vi "PicoReadPicoMultiBuffers.vi"(1 "enabled array":i16[](array[numeric]), 2 "Buffer and Transfer Settings":T3={"startIndex"=0, "Samples"=1000000, "Down Sample Ratio"=1, "Down-Sample Mode"=2147483648} {"Down-Sample Mode" items=["None"=2147483648, "Aggregate"=1, "Decimate"=2, "Average"=4]; "Down Sample Ratio" step=1; "Samples" format="%_6p"}, 3 "Variant":string, 5 "Data Pointers":T1, 9 "No of Buffers":i32=1, 11 "error in (no error)":errorcluster) -> (6 "MultiBuffers (Max or non-aggregated)":T2(array[cluster]), 8 "Min Buffers":T2(array[cluster]), 15 "error out":errorcluster)   [LabVIEW 2020]
doc: "Read data from Picodata buffers for Block and 6000a streaming examples"
uses:
  PicoBuffers.ctl
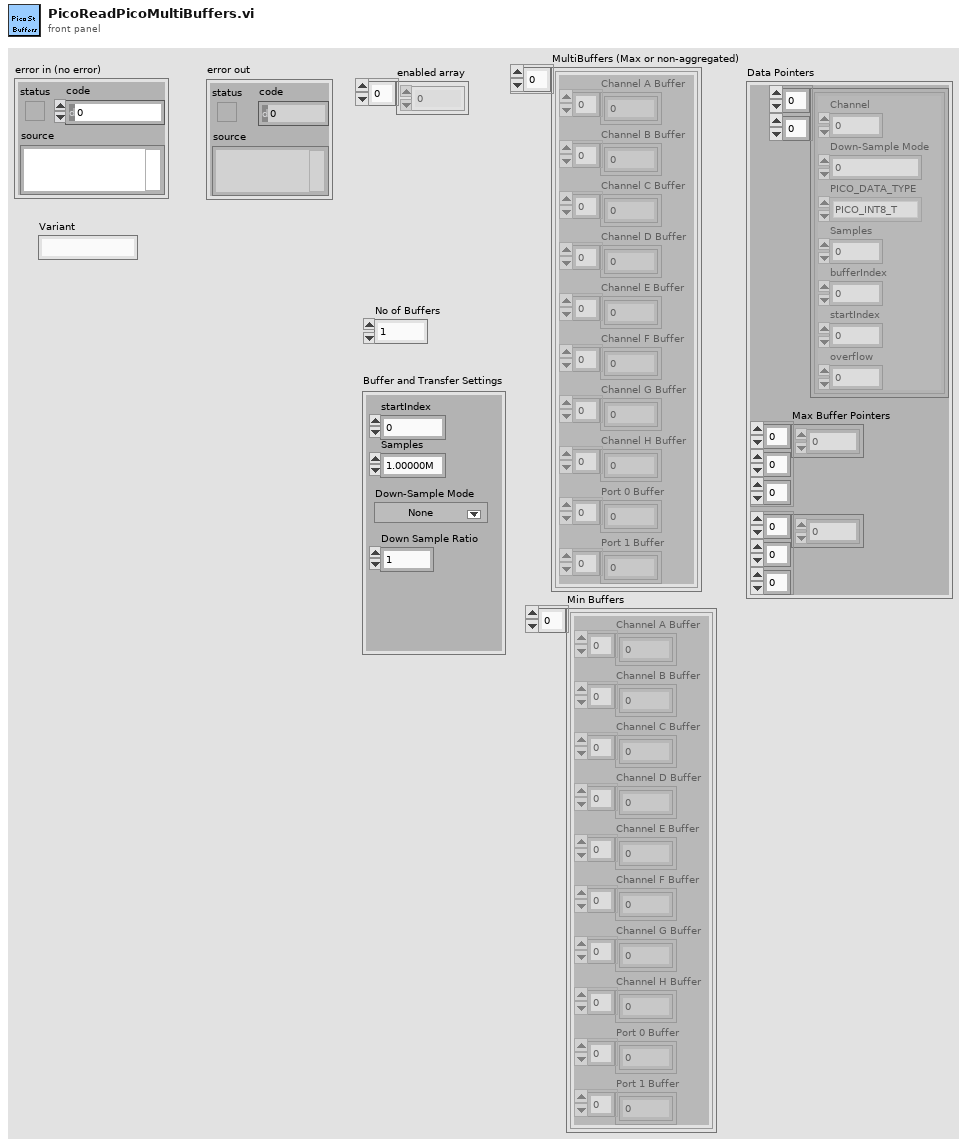
[diagram p1: front panel]
types:
  T1 = typedef "PicoBuffers.ctl" = cluster{"Max Buffer Pointers":u64[][][], "Min Buffer Pointers":u64[][][], "StreamingDataInfo":cluster{"Channel":u32, "Down-Sample Mode":u32, "PICO_DATA_TYPE":enum32{"PICO_INT8_T", "PICO_INT16_T", "PICO_INT32_T", "PICO_UINT32_T", "PICO_INT64_T", ""}, "Samples":i32, "bufferIndex":u64, "startIndex":i32, "overflow":i16}[][]}
  T2 = cluster{"Channel A Buffer":i16[], "Channel B Buffer":i16[], "Channel C Buffer":i16[], "Channel D Buffer":i16[], "Channel E Buffer":i16[], "Channel F Buffer":i16[], "Channel G Buffer":i16[], "Channel H Buffer":i16[], "Port 0 Buffer":i16[], "Port 1 Buffer":i16[]}[]
  T3 = cluster{"startIndex":u64, "Samples":u64, "Down Sample Ratio":u64, "Down-Sample Mode":u32}
  T4 = cluster{"Channel A Buffer":i16[], "Channel B Buffer":i16[], "Channel C Buffer":i16[], "Channel D Buffer":i16[], "Channel E Buffer":i16[], "Channel F Buffer":i16[], "Channel G Buffer":i16[], "Channel H Buffer":i16[], "Port 0 Buffer":i16[], "Port 1 Buffer":i16[]}
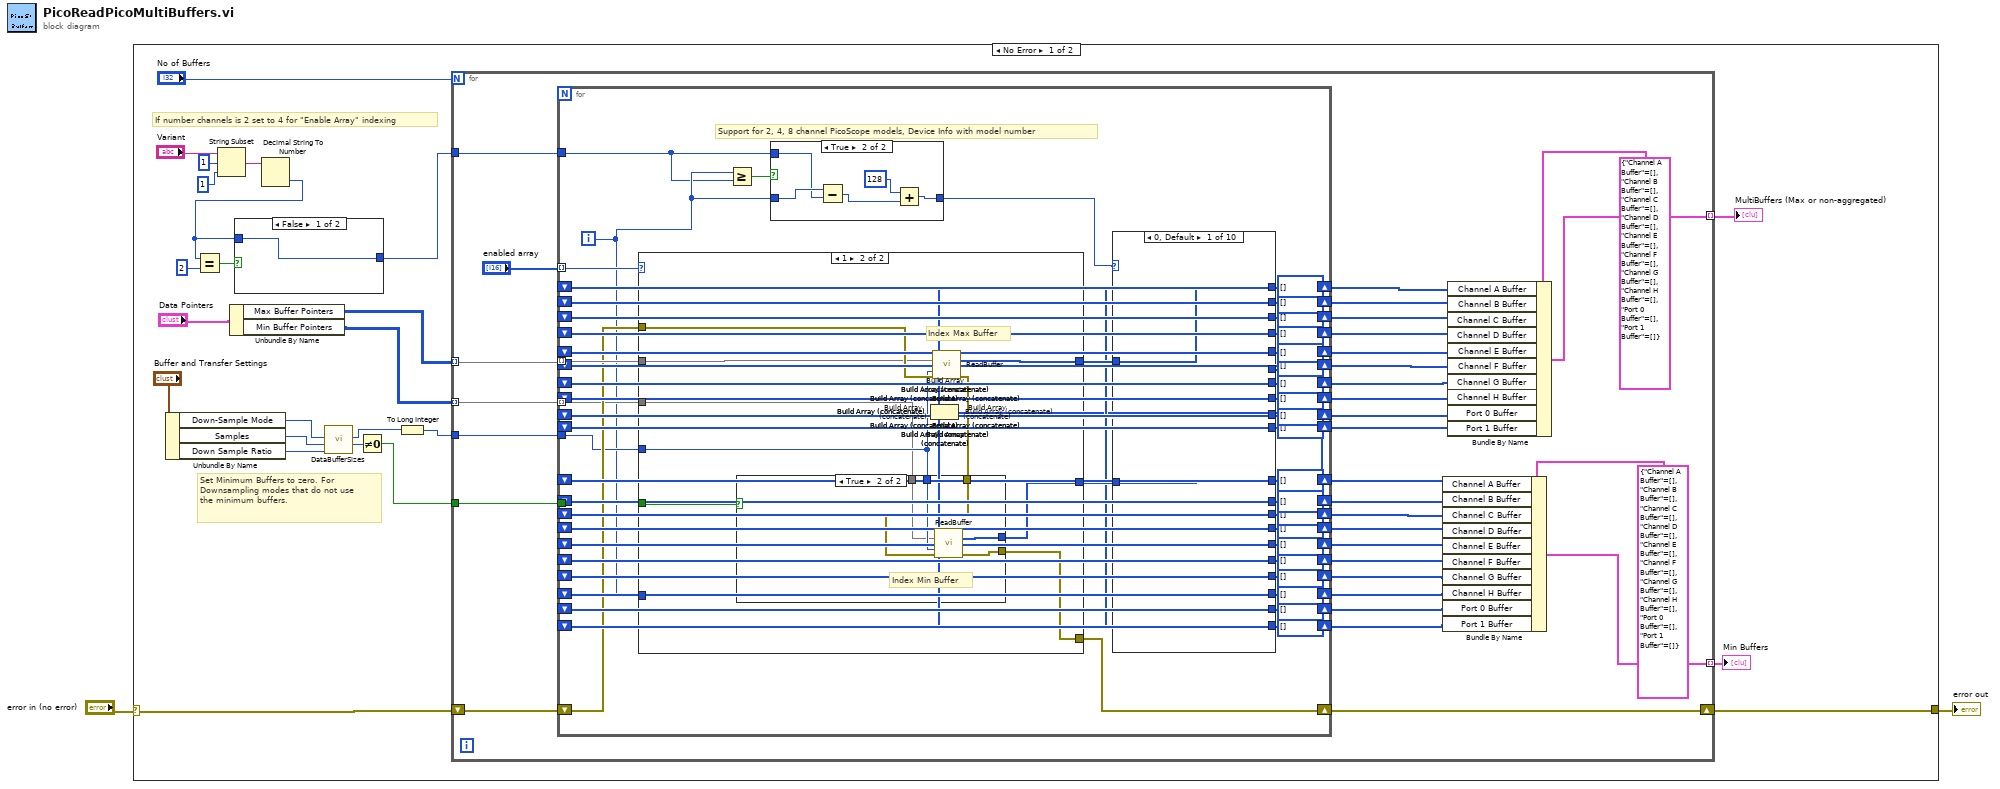
[diagram p0: block diagram]
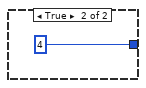
[diagram p2: hidden frame]
diagram:
  n1 = case shown="No Error" "error in (no error)" {
    selector: "error in (no error)" -> [w24 w196]
    tunnel: [w26 w196] -> w1
    frame No Error {
      # "If number channels is 2 set to 4 for \"Enable Array\" indexing"
      # "Set Minimum Buffers to zero. For Downsampling modes that do not use the minimum buffers."
      n2 = Unbundle By Name("Buffer and Transfer Settings") -> ("Down-Sample Mode"=w22:u32, "Samples"=w21:u64, "Down Sample Ratio"=w23:u64)
      n3 = String Subset(string="Variant", offset (0)=1, length (rest)=1 ("length (rest)")) -> (substring=w7:string)
      n4 = Unbundle By Name("Data Pointers") -> ("Max Buffer Pointers"=w12:u64[][][], "Min Buffer Pointers"=w11:u64[][][])
      n5 = Decimal String To Number(string=w7) -> (number=w4:i32)  [unwired: 2 in, 1 out]
      n6 = Equal?(x=w4, y=2 ("Number of channels")) -> (x = y?=w10:bool)
      n7 = case shown="False" w10 {
        tunnel: [w27 4 ("Number of channels")] -> w8
        tunnel: w4 -> [w27 _]
        frame False {
        }
        frame True {
        }
      }
      n8 = call "DataBufferSizes.vi"("Down Sample Ratio"=w23, "Number of Samples"=w21, "Down-Sample Mode"=w22) -> ("min Buffer Size"=w19:i32, "Max Buffer Size"=w15:i32)  [unwired: 7 in]
      n9 = Not Equal To 0?(x=w19) -> (x != 0?=w20:bool)
      n10 = To Long Integer(number=w15) -> (32bit integer=w18:i32)
      n11 = for {
        N: "No of Buffers" -> [_]
        tunnel: [w78] -> w14 mode=indexing
        tunnel: [w77] -> w16 mode=indexing
        tunnel: w20 -> [w65]
        tunnel: w18 -> [w63]
        shift-right: [w80] -> w26
        shift-left: w24 -> [w79]
        tunnel: w12 -> [w61] mode=indexing
        tunnel: w11 -> [w50] mode=indexing
        tunnel: w8 -> [w49]
        n12 = for {
          tunnel: "enabled array" -> [w152] mode=indexing
          tunnel: w61 -> [w153] mode=indexing
          shift-right: [w151] -> w80
          shift-left: w79 -> [w150]
          tunnel: w63 -> [w136]
          tunnel: w65 -> [w135]
          tunnel: w50 -> [w125] mode=indexing
          tunnel: w49 -> [w121]
          shift-right: [w119] -> w76
          shift-left: i16[] [] ("Output Array") -> [w120]
          shift-right: [w117] -> w75
          shift-left: i16[] [] ("Output Array") -> [w118]
          shift-right: [w115] -> w74
          shift-left: i16[] [] ("Output Array") -> [w116]
          shift-right: [w113] -> w73
          shift-left: i16[] [] ("Output Array") -> [w114]
          shift-right: [w111] -> w72
          shift-left: i16[] [] ("Output Array") -> [w112]
          shift-right: [w109] -> w71
          shift-left: i16[] [] ("Output Array") -> [w110]
          shift-right: [w107] -> w64
          shift-left: i16[] [] ("Output Array") -> [w108]
          shift-right: [w105] -> w70
          shift-left: i16[] [] ("Output Array") -> [w106]
          shift-right: [w103] -> w69
          shift-left: i16[] [] ("Output Array") -> [w104]
          shift-right: [w101] -> w68
          shift-left: i16[] [] ("Output Array") -> [w102]
          shift-right: [w99] -> w67
          shift-left: i16[] [] ("Output Array") -> [w100]
          shift-right: [w97] -> w66
          shift-left: i16[] [] ("Output Array") -> [w98]
          shift-right: [w95] -> w58
          shift-left: i16[] [] ("Output Array") -> [w96]
          shift-right: [w93] -> w57
          shift-left: i16[] [] ("Output Array") -> [w94]
          shift-right: [w91] -> w56
          shift-left: i16[] [] ("Output Array") -> [w92]
          shift-right: [w89] -> w55
          shift-left: i16[] [] ("Output Array") -> [w90]
          shift-right: [w87] -> w54
          shift-left: i16[] [] ("Output Array") -> [w88]
          shift-right: [w85] -> w53
          shift-left: i16[] [] ("Output Array") -> [w86]
          shift-right: [w83] -> w52
          shift-left: i16[] [] ("Output Array") -> [w84]
          shift-right: [w81] -> w51
          shift-left: i16[] [] ("Output Array") -> [w82]
          i -> [w122]
          # "Support for 2, 4, 8 channel PicoScope models, Device Info with model number"
          n13 = case shown="1" w152 {
            tunnel: w153 -> [_ w182]
            tunnel: w122 -> [_ _]
            tunnel: [_ w189] -> w149
            tunnel: [_ w188] -> w148
            tunnel: w150 -> [w180 w187]
            tunnel: [w180 w185] -> w151
            tunnel: w136 -> [_ w183]
            tunnel: w135 -> [_ w184]
            tunnel: w125 -> [_ w181]
            frame 0, Default {
            }
            frame 1 {
              # "Index Max Buffer"
              n14 = call "ReadBuffer.vi"("Pointer and BufferSize"=w182, "Buffer size"=w183, "error in (no error)"=w187) -> ("Output Array"=w189:i16[], "error out"=w186:errorcluster)  [unwired: 11 in]
              n15 = case shown="True" w184 {
                tunnel: [_ w195] -> w188
                tunnel: w186 -> [w190 w194]
                tunnel: [w190 w193] -> w185
                tunnel: w183 -> [_ w192]
                tunnel: w181 -> [_ w191]
                frame False {
                }
                frame True {
                  # "Index Min Buffer"
                  n16 = call "ReadBuffer.vi"("Pointer and BufferSize"=w191, "Buffer size"=w192, "error in (no error)"=w194) -> ("Output Array"=w195:i16[], "error out"=w193:errorcluster)  [unwired: 11 in]
                }
              }
            }
          }
          n17 = Greater Or Equal?(x=w122, y=w121) -> (x >= y?=w124:bool)
          n18 = case shown="True" w124 {
            tunnel: w122 -> [w154 w156]
            tunnel: [w154 w158] -> w123
            tunnel: w121 -> [_ w155]
            frame False {
            }
            frame True {
              n19 = Subtract(x=w156, y=w155) -> (x-y=w157:i32)
              n20 = Add(x=128, y=w157) -> (x+y=w158:i32)
            }
          }
          n21 = case shown="0, Default" w123 {
            tunnel: w149 -> [w161 w163 w165 w167 w169 w171 w173 w175 w177 w179]
            tunnel: [w161 _ _ _ _ _ _ _ _ _] -> w134
            tunnel: [_ w163 _ _ _ _ _ _ _ _] -> w141
            tunnel: [_ _ w165 _ _ _ _ _ _ _] -> w140
            tunnel: [_ _ _ w167 _ _ _ _ _ _] -> w139
            tunnel: [_ _ _ _ w169 _ _ _ _ _] -> w138
            tunnel: [_ _ _ _ _ w171 _ _ _ _] -> w137
            tunnel: w148 -> [w160 w162 w164 w166 w168 w170 w172 w174 w176 w178]
            tunnel: [w160 _ _ _ _ _ _ _ _ _] -> w147
            tunnel: [_ w162 _ _ _ _ _ _ _ _] -> w146
            tunnel: [_ _ w164 _ _ _ _ _ _ _] -> w145
            tunnel: [_ _ _ w166 _ _ _ _ _ _] -> w144
            tunnel: [_ _ _ _ w168 _ _ _ _ _] -> w143
            tunnel: [_ _ _ _ _ w170 _ _ _ _] -> w142
            tunnel: [_ _ _ _ _ _ w173 _ _ _] -> w133
            tunnel: [_ _ _ _ _ _ w172 _ _ _] -> w132
            tunnel: [_ _ _ _ _ _ _ w175 _ _] -> w131
            tunnel: [_ _ _ _ _ _ _ w174 _ _] -> w130
            tunnel: [_ _ _ _ _ _ _ _ w177 _] -> w129
            tunnel: [_ _ _ _ _ _ _ _ w176 _] -> w128
            tunnel: [_ _ _ _ _ _ _ _ _ w179] -> w127
            tunnel: [_ _ _ _ _ _ _ _ _ w178] -> w126
            frame 0, Default {
            }
            frame 1 {
            }
            frame 2 {
            }
            frame 3 {
            }
            frame 4 {
            }
            frame 5 {
            }
            frame 6 {
            }
            frame 7 {
            }
            frame 128 {
            }
            frame 129 {
            }
          }
          n22 = Build Array (concatenate)(w82, w126) -> (w81:i16[])
          n23 = Build Array (concatenate)(w84, w127) -> (w83:i16[])
          n24 = Build Array (concatenate)(w86, w128) -> (w85:i16[])
          n25 = Build Array (concatenate)(w88, w129) -> (w87:i16[])
          n26 = Build Array (concatenate)(w90, w130) -> (w89:i16[])
          n27 = Build Array (concatenate)(w92, w131) -> (w91:i16[])
          n28 = Build Array (concatenate)(w94, w132) -> (w93:i16[])
          n29 = Build Array (concatenate)(w96, w133) -> (w95:i16[])
          n30 = Build Array (concatenate)(w98, w137) -> (w97:i16[])
          n31 = Build Array (concatenate)(w100, w138) -> (w99:i16[])
          n32 = Build Array (concatenate)(w102, w139) -> (w101:i16[])
          n33 = Build Array (concatenate)(w104, w140) -> (w103:i16[])
          n34 = Build Array (concatenate)(w106, w141) -> (w105:i16[])
          n35 = Build Array (concatenate)(w108, w134) -> (w107:i16[])
          n36 = Build Array (concatenate)(w110, w142) -> (w109:i16[])
          n37 = Build Array (concatenate)(w112, w143) -> (w111:i16[])
          n38 = Build Array (concatenate)(w114, w144) -> (w113:i16[])
          n39 = Build Array (concatenate)(w116, w145) -> (w115:i16[])
          n40 = Build Array (concatenate)(w118, w146) -> (w117:i16[])
          n41 = Build Array (concatenate)(w120, w147) -> (w119:i16[])
        }
        n42 = Bundle By Name(cluster=T4 {"Channel A Buffer"=[], "Channel B Buffer"=[], "Channel C Buffer"=[], "Channel D Buffer"=[], "Channel E Buffer"=[], "Channel F Buffer"=[], "Channel G Buffer"=[], "Channel H Buffer"=[], "Port 0 Buffer"=[], "Port 1 Buffer"=[]} ("input cluster"), "Channel A Buffer"=w76, "Channel B Buffer"=w75, "Channel C Buffer"=w74, "Channel D Buffer"=w73, "Channel E Buffer"=w72, "Channel F Buffer"=w71, "Channel G Buffer"=w57, "Channel H Buffer"=w55, "Port 0 Buffer"=w53, "Port 1 Buffer"=w51) -> (w78:T4)
        n43 = Bundle By Name(cluster=T4 {"Channel A Buffer"=[], "Channel B Buffer"=[], "Channel C Buffer"=[], "Channel D Buffer"=[], "Channel E Buffer"=[], "Channel F Buffer"=[], "Channel G Buffer"=[], "Channel H Buffer"=[], "Port 0 Buffer"=[], "Port 1 Buffer"=[]} ("input cluster"), "Channel A Buffer"=w64, "Channel B Buffer"=w70, "Channel C Buffer"=w69, "Channel D Buffer"=w68, "Channel E Buffer"=w67, "Channel F Buffer"=w66, "Channel G Buffer"=w58, "Channel H Buffer"=w56, "Port 0 Buffer"=w54, "Port 1 Buffer"=w52) -> (w77:T4)
      }
      "MultiBuffers (Max or non-aggregated)" <- w16
      "Min Buffers" <- w14
    }
    frame Error {
    }
  }
  "error out" <- w1
